vi "Dequeue Item.vi"(8 "error in (no error)":errorcluster, 11 "Queue in":refnum<queue>) -> (0 "error out":errorcluster, 1 "Variant":variant, 2 "String":string, 3 "Queue out":refnum<queue>)   [LabVIEW 2017]
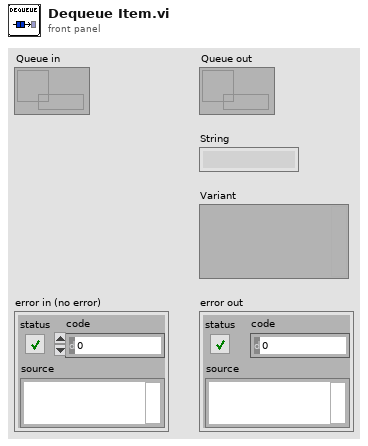
[diagram p1: front panel]
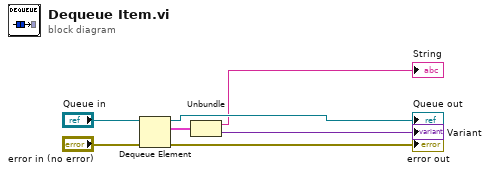
[diagram p0: block diagram]
diagram:
  n1 = Dequeue Element(queue="Queue in", error in (no error)="error in (no error)") -> (queue out=→"Queue out":refnum<queue>, element=w3:cluster{string, variant}, error out=→"error out":errorcluster)  [unwired: 1 in, 1 out]
  n2 = Unbundle(w3) -> (→"String":string, →"Variant":variant)
